vi "lvstyx_get_dirent_name.vi"(2 "error in (no error)":errorcluster, 5 "dirent ptr":u32) -> (0 "error out":errorcluster, 1 "name":string)   [LabVIEW 2010, in "lib1299.lvlib"]
uses:
  lib1299.lvlib
  cstyx/win32/cstyx.dll
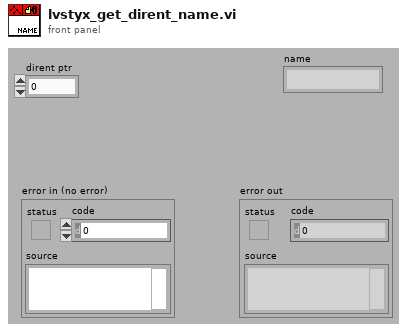
[diagram p1: front panel]
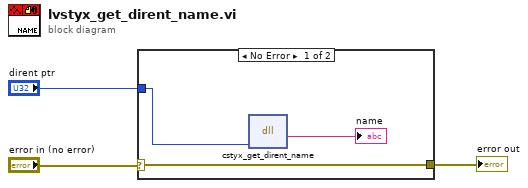
[diagram p0: block diagram]
diagram:
  n1 = case shown="No Error" "error in (no error)" {
    selector: "error in (no error)" -> [w4 w7]
    tunnel: "dirent ptr" -> [w6 _]
    tunnel: [w4 w7] -> w2
    frame No Error {
      n2 = dll-call lib="C:/work/ads1299evm/lib_1299/Styx/cstyx/win32/cstyx.dll" fn="cstyx_get_dirent_name"("dirent"=w6) -> ("name"=→"name":string)  [unwired: 4 in, 2 out]
    }
    frame Error {
    }
  }
  "error out" <- w2
